vi "SP Convert Marker Types to Frequencies.vi"(4 "CH 2":T1, 5 "CH 1":T1, 8 "Marker":T2) -> (0 "CH2 Index":i32, 1 "CH2 Frequency":dbl, 2 "CH1 Index":i32, 3 "CH1 Frequency":dbl)   [LabVIEW 2011]
uses:
  TypeDefs/SP Marker Cluster.ctl
  TypeDefs/SP Marker Type.ctl
  TypeDefs/SP Channel Data.ctl
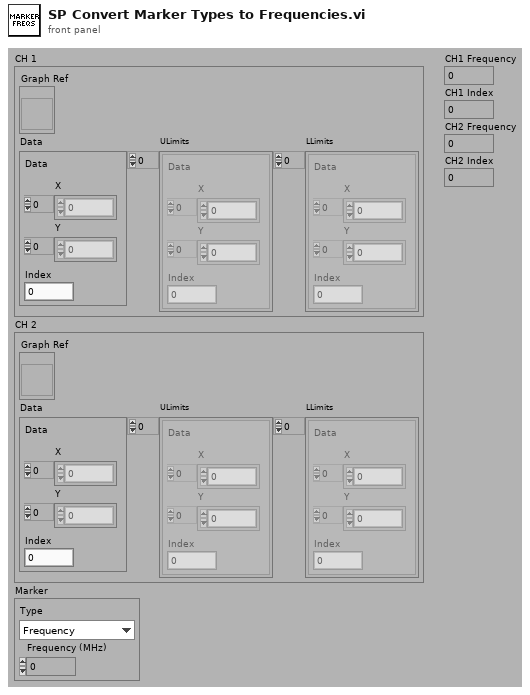
[diagram p1: front panel]
types:
  T1 = typedef "SP Channel Data.ctl" = cluster{"Graph Ref":refnum<vi>, "Data":cluster{"Data":cluster{"X":dbl[], "Y":dbl[]}, "Index":i32}, "ULimits":cluster{"Data":cluster{"X":dbl[], "Y":dbl[]}, "Index":i32}[], "LLimits":cluster{"Data":cluster{"X":dbl[], "Y":dbl[]}, "Index":i32}[]}
  T2 = typedef "SP Marker Cluster.ctl" = cluster{"Type":T3, "Frequency (MHz)":dbl}
  T3 = typedef "SP Marker Type.ctl" = enum16{"Frequency", "Trace Maximum", "Trace Minimum", "Limit Maximum", "Limit Minimum"}
  T4 = cluster{"Data":cluster{"X":dbl[], "Y":dbl[]}, "Index":i32}[]
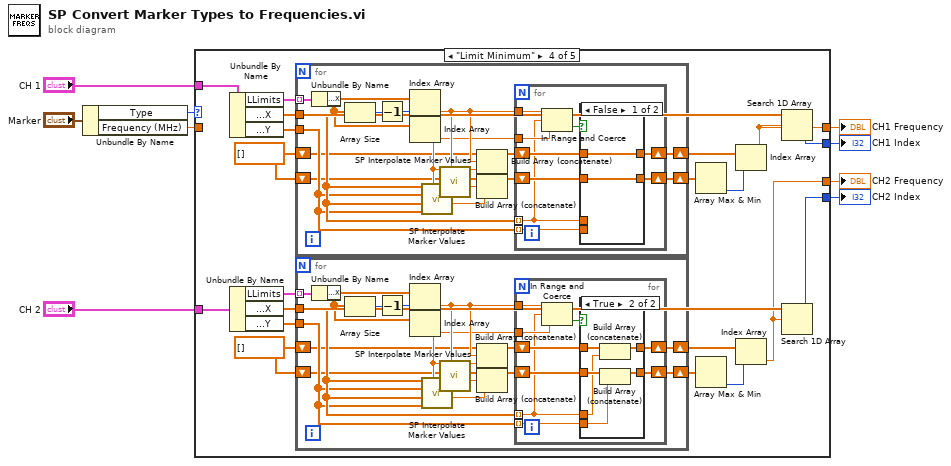
[diagram p0: block diagram]
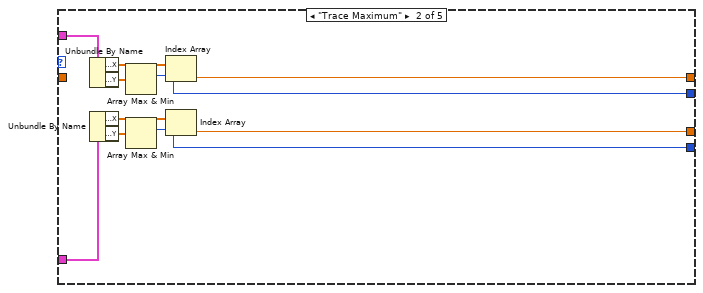
[diagram p3: hidden frame]
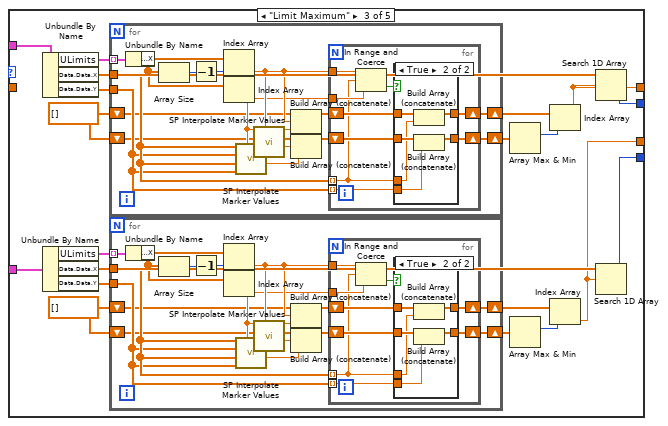
[diagram p4: hidden frame]
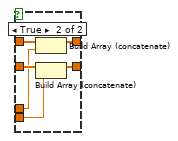
[diagram p8: hidden frame]
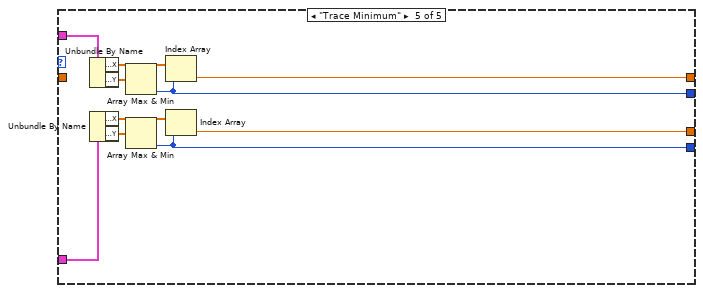
[diagram p9: hidden frame]
diagram:
  n1 = Unbundle By Name("Marker") -> ("Type"=w4:T3, "Frequency (MHz)"=w3:dbl)
  n2 = case shown="\"Limit Minimum\"" w4 {
    tunnel: w3 -> [w10 _ _ _ _]
    tunnel: [w10 w16 w23 w112 w198] -> w8
    tunnel: "CH 1" -> [_ w13 w29 w115 w195]
    tunnel: "CH 2" -> [_ w14 w30 w116 w196]
    tunnel: [w10 w15 w27 w109 w197] -> w7
    tunnel: [_ w12 w25 w108 w193] -> w2
    tunnel: [_ w11 w21 w107 w194] -> w1
    frame "Frequency", Default {
    }
    frame "Trace Maximum" {
      n3 = Unbundle By Name(w13) -> ("Data.Data.X"=w19:dbl[], "Data.Data.Y"=w20:dbl[])
      n4 = Unbundle By Name(w14) -> ("Data.Data.X"=w18:dbl[], "Data.Data.Y"=w17:dbl[])
      n5 = Array Max & Min(array=w20) -> (max index (indices)=w11:i32)  [unwired: 3 out]
      n6 = Array Max & Min(array=w17) -> (max index (indices)=w12:i32)  [unwired: 3 out]
      n7 = Index Array(array=w19, index=w11) -> (element=w16:dbl)
      n8 = Index Array(array=w18, index=w12) -> (element=w15:dbl)
    }
    frame "Limit Maximum" {
      w33 = dbl[] []
      w38 = dbl[] []
      n9 = Unbundle By Name(w29) -> ("ULimits"=w40:T4, "Data.Data.X"=w24:dbl[], "Data.Data.Y"=w39:dbl[])
      n10 = Unbundle By Name(w30) -> ("ULimits"=w31:T4, "Data.Data.X"=w28:dbl[], "Data.Data.Y"=w32:dbl[])
      n11 = for {
        tunnel: w40 -> [w89] mode=indexing
        tunnel: w24 -> [w83]
        tunnel: w39 -> [w82]
        shift-right: [w79] -> w36
        shift-left: w38 -> [w77]
        shift-right: [w78] -> w37
        shift-left: w38 -> [w75]
        n12 = Unbundle By Name(w89) -> ("Data.X"=w84:dbl[])
        n13 = Array Size(array=w84) -> (size(s)=w88:i32)
        n14 = Decrement(x=w88) -> (x-1=w85:i32)
        n15 = Index Array(array=w84, index=w85) -> (element=w81:dbl)
        n16 = Index Array(array=w84) -> (element=w80:dbl)  [unwired: 1 in]
        n17 = call "SP Interpolate Marker Values.vi"("Marker Value"=w80, "Y Values"=w82, "X Values"=w83) -> ("Interpolated Y Value"=w86:dbl)  [unwired: 8 out]
        n18 = call "SP Interpolate Marker Values.vi"("Marker Value"=w81, "Y Values"=w82, "X Values"=w83) -> ("Interpolated Y Value"=w87:dbl)  [unwired: 8 out]
        n19 = Build Array (concatenate)(w77, w81, w80) -> (w76:dbl[])
        n20 = Build Array (concatenate)(w75, w87, w86) -> (w74:dbl[])
        n21 = for {
          tunnel: w81 -> [w98]
          tunnel: w80 -> [w97]
          tunnel: w83 -> [w90] mode=indexing
          tunnel: w82 -> [w93] mode=indexing
          shift-right: [w94] -> w78
          shift-left: w74 -> [w95]
          shift-right: [w91] -> w79
          shift-left: w76 -> [w92]
          n22 = In Range and Coerce(upper limit=w98, x=w90, lower limit=w97) -> (In Range?=w96:bool)  [unwired: 1 out]
          n23 = case shown="True" w96 {
            tunnel: w95 -> [w100 w106]
            tunnel: [w100 w105] -> w94
            tunnel: w93 -> [_ w104]
            tunnel: w92 -> [w99 w103]
            tunnel: [w99 w102] -> w91
            tunnel: w90 -> [_ w101]
            frame False {
            }
            frame True {
              n24 = Build Array (concatenate)(w103, w101) -> (w102:dbl[])
              n25 = Build Array (concatenate)(w106, w104) -> (w105:dbl[])
            }
          }
        }
      }
      n26 = for {
        tunnel: w31 -> [w56] mode=indexing
        tunnel: w28 -> [w50]
        tunnel: w32 -> [w49]
        shift-right: [w46] -> w35
        shift-left: w33 -> [w44]
        shift-right: [w45] -> w34
        shift-left: w33 -> [w42]
        n27 = Unbundle By Name(w56) -> ("Data.X"=w51:dbl[])
        n28 = Array Size(array=w51) -> (size(s)=w55:i32)
        n29 = Decrement(x=w55) -> (x-1=w52:i32)
        n30 = Index Array(array=w51, index=w52) -> (element=w48:dbl)
        n31 = Index Array(array=w51) -> (element=w47:dbl)  [unwired: 1 in]
        n32 = call "SP Interpolate Marker Values.vi"("Marker Value"=w47, "Y Values"=w49, "X Values"=w50) -> ("Interpolated Y Value"=w53:dbl)  [unwired: 8 out]
        n33 = call "SP Interpolate Marker Values.vi"("Marker Value"=w48, "Y Values"=w49, "X Values"=w50) -> ("Interpolated Y Value"=w54:dbl)  [unwired: 8 out]
        n34 = Build Array (concatenate)(w44, w48, w47) -> (w43:dbl[])
        n35 = Build Array (concatenate)(w42, w54, w53) -> (w41:dbl[])
        n36 = for {
          tunnel: w48 -> [w65]
          tunnel: w47 -> [w64]
          tunnel: w50 -> [w57] mode=indexing
          tunnel: w49 -> [w60] mode=indexing
          shift-right: [w61] -> w45
          shift-left: w41 -> [w62]
          shift-right: [w58] -> w46
          shift-left: w43 -> [w59]
          n37 = In Range and Coerce(upper limit=w65, x=w57, lower limit=w64) -> (In Range?=w63:bool)  [unwired: 1 out]
          n38 = case shown="True" w63 {
            tunnel: w62 -> [w67 w73]
            tunnel: [w67 w72] -> w61
            tunnel: w60 -> [_ w71]
            tunnel: w59 -> [w66 w70]
            tunnel: [w66 w69] -> w58
            tunnel: w57 -> [_ w68]
            frame False {
            }
            frame True {
              n39 = Build Array (concatenate)(w70, w68) -> (w69:dbl[])
              n40 = Build Array (concatenate)(w73, w71) -> (w72:dbl[])
            }
          }
        }
      }
      n41 = Array Max & Min(array=w37) -> (max index (indices)=w22:i32)  [unwired: 3 out]
      n42 = Array Max & Min(array=w34) -> (max index (indices)=w26:i32)  [unwired: 3 out]
      n43 = Index Array(array=w36, index=w22) -> (element=w23:dbl)
      n44 = Index Array(array=w35, index=w26) -> (element=w27:dbl)
      n45 = Search 1D Array(1D array=w24, element=w23) -> (index of element=w21:i32)  [unwired: 1 out]
      n46 = Search 1D Array(1D array=w28, element=w27) -> (index of element=w25:i32)  [unwired: 1 out]
    }
    frame "Limit Minimum" {
      w119 = dbl[] []
      w124 = dbl[] []
      n47 = Unbundle By Name(w115) -> ("LLimits"=w126:T4, "Data.Data.X"=w113:dbl[], "Data.Data.Y"=w125:dbl[])
      n48 = Unbundle By Name(w116) -> ("LLimits"=w117:T4, "Data.Data.X"=w114:dbl[], "Data.Data.Y"=w118:dbl[])
      n49 = for {
        tunnel: w126 -> [w175] mode=indexing
        tunnel: w113 -> [w169]
        tunnel: w125 -> [w168]
        shift-right: [w165] -> w122
        shift-left: w124 -> [w163]
        shift-right: [w164] -> w123
        shift-left: w124 -> [w161]
        n50 = Unbundle By Name(w175) -> ("Data.X"=w170:dbl[])
        n51 = Array Size(array=w170) -> (size(s)=w174:i32)
        n52 = Decrement(x=w174) -> (x-1=w171:i32)
        n53 = Index Array(array=w170, index=w171) -> (element=w167:dbl)
        n54 = Index Array(array=w170) -> (element=w166:dbl)  [unwired: 1 in]
        n55 = call "SP Interpolate Marker Values.vi"("Marker Value"=w166, "Y Values"=w168, "X Values"=w169) -> ("Interpolated Y Value"=w172:dbl)  [unwired: 8 out]
        n56 = call "SP Interpolate Marker Values.vi"("Marker Value"=w167, "Y Values"=w168, "X Values"=w169) -> ("Interpolated Y Value"=w173:dbl)  [unwired: 8 out]
        n57 = Build Array (concatenate)(w163, w167, w166) -> (w162:dbl[])
        n58 = Build Array (concatenate)(w161, w173, w172) -> (w160:dbl[])
        n59 = for {
          tunnel: w167 -> [w184]
          tunnel: w166 -> [w183]
          tunnel: w169 -> [w176] mode=indexing
          tunnel: w168 -> [w179] mode=indexing
          shift-right: [w180] -> w164
          shift-left: w160 -> [w181]
          shift-right: [w177] -> w165
          shift-left: w162 -> [w178]
          n60 = In Range and Coerce(upper limit=w184, x=w176, lower limit=w183) -> (In Range?=w182:bool)  [unwired: 1 out]
          n61 = case shown="False" w182 {
            tunnel: w181 -> [w186 w192]
            tunnel: [w186 w191] -> w180
            tunnel: w179 -> [_ w190]
            tunnel: w178 -> [w185 w189]
            tunnel: [w185 w188] -> w177
            tunnel: w176 -> [_ w187]
            frame False {
            }
            frame True {
              n62 = Build Array (concatenate)(w189, w187) -> (w188:dbl[])
              n63 = Build Array (concatenate)(w192, w190) -> (w191:dbl[])
            }
          }
        }
      }
      n64 = for {
        tunnel: w117 -> [w142] mode=indexing
        tunnel: w114 -> [w136]
        tunnel: w118 -> [w135]
        shift-right: [w132] -> w121
        shift-left: w119 -> [w130]
        shift-right: [w131] -> w120
        shift-left: w119 -> [w128]
        n65 = Unbundle By Name(w142) -> ("Data.X"=w137:dbl[])
        n66 = Array Size(array=w137) -> (size(s)=w141:i32)
        n67 = Decrement(x=w141) -> (x-1=w138:i32)
        n68 = Index Array(array=w137, index=w138) -> (element=w134:dbl)
        n69 = Index Array(array=w137) -> (element=w133:dbl)  [unwired: 1 in]
        n70 = call "SP Interpolate Marker Values.vi"("Marker Value"=w133, "Y Values"=w135, "X Values"=w136) -> ("Interpolated Y Value"=w139:dbl)  [unwired: 8 out]
        n71 = call "SP Interpolate Marker Values.vi"("Marker Value"=w134, "Y Values"=w135, "X Values"=w136) -> ("Interpolated Y Value"=w140:dbl)  [unwired: 8 out]
        n72 = Build Array (concatenate)(w130, w134, w133) -> (w129:dbl[])
        n73 = Build Array (concatenate)(w128, w140, w139) -> (w127:dbl[])
        n74 = for {
          tunnel: w134 -> [w151]
          tunnel: w133 -> [w150]
          tunnel: w136 -> [w143] mode=indexing
          tunnel: w135 -> [w146] mode=indexing
          shift-right: [w147] -> w131
          shift-left: w127 -> [w148]
          shift-right: [w144] -> w132
          shift-left: w129 -> [w145]
          n75 = In Range and Coerce(upper limit=w151, x=w143, lower limit=w150) -> (In Range?=w149:bool)  [unwired: 1 out]
          n76 = case shown="True" w149 {
            tunnel: w148 -> [w153 w159]
            tunnel: [w153 w158] -> w147
            tunnel: w146 -> [_ w157]
            tunnel: w145 -> [w152 w156]
            tunnel: [w152 w155] -> w144
            tunnel: w143 -> [_ w154]
            frame False {
            }
            frame True {
              n77 = Build Array (concatenate)(w156, w154) -> (w155:dbl[])
              n78 = Build Array (concatenate)(w159, w157) -> (w158:dbl[])
            }
          }
        }
      }
      n79 = Array Max & Min(array=w123) -> (min index (indices)=w111:i32)  [unwired: 3 out]
      n80 = Array Max & Min(array=w120) -> (min index (indices)=w110:i32)  [unwired: 3 out]
      n81 = Index Array(array=w122, index=w111) -> (element=w112:dbl)
      n82 = Index Array(array=w121, index=w110) -> (element=w109:dbl)
      n83 = Search 1D Array(1D array=w113, element=w112) -> (index of element=w107:i32)  [unwired: 1 out]
      n84 = Search 1D Array(1D array=w114, element=w109) -> (index of element=w108:i32)  [unwired: 1 out]
    }
    frame "Trace Minimum" {
      n85 = Unbundle By Name(w195) -> ("Data.Data.X"=w201:dbl[], "Data.Data.Y"=w202:dbl[])
      n86 = Unbundle By Name(w196) -> ("Data.Data.X"=w200:dbl[], "Data.Data.Y"=w199:dbl[])
      n87 = Array Max & Min(array=w202) -> (min index (indices)=w194:i32)  [unwired: 3 out]
      n88 = Array Max & Min(array=w199) -> (min index (indices)=w193:i32)  [unwired: 3 out]
      n89 = Index Array(array=w201, index=w194) -> (element=w198:dbl)
      n90 = Index Array(array=w200, index=w193) -> (element=w197:dbl)
    }
  }
  "CH1 Frequency" <- w8
  "CH2 Frequency" <- w7
  "CH1 Index" <- w1
  "CH2 Index" <- w2
